vi "Create Gradient 32f.vi"(8 "Error In":errorcluster, 9 "Dimension":T1={"Depth"=1, "Height"=1, "Width"=1} {"Width" min=1; "Height" min=1; "Depth" min=1}, 11 "Device In":T4) -> (0 "Error Out":errorcluster, 1 "Dimension Out":T1={"Depth"=1, "Height"=1, "Width"=1} {"Width" min=1; "Height" min=1; "Depth" min=1}, 3 "Gradient Object":T2 {"Z"."Dimension"."Width" min=1; "Z"."Dimension"."Height" min=1; "Z"."Dimension"."Depth" min=1; "Y"."Dimension"."Width" min=1; "Y"."Dimension"."Height" min=1; "Y"."Dimension"."Depth" min=1; "X"."Dimension"."Width" min=1; "X"."Dimension"."Height" min=1; "X"."Dimension"."Depth" min=1})   [LabVIEW 2012, in "OpenCLV x64.lvlib"]
doc: "Creates a Gradient Object and allocates space for an X, Y, and Z destination memory objects."
uses:
  OpenCLV x64.lvlib
  Controls/Device ID.ctl
  User Controls/Array Dimensions.ctl
  Controls/Gradient Object.ctl
  Controls/Program Handle.ctl
  Controls/Memory Object.ctl
  Controls/Memory ID.ctl
  Controls/Memory Type.ctl
  Allocate Memory/AllocateMemory_32f.vi
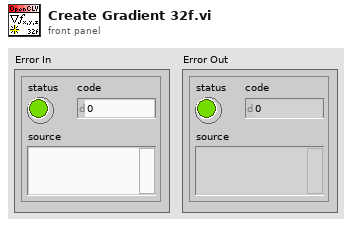
[diagram p1: front panel]
types:
  T1 = typedef "Array Dimensions.ctl" = cluster{"Depth":u64, "Height":u64, "Width":u64}
  T2 = typedef "OpenCLV x64.lvlib/Gradient Object.ctl" = cluster{"Program Handle":T3, "Device Out":T4, "X":T5, "Y":T5, "Z":T5}
  T3 = typedef "OpenCLV x64.lvlib/Program Handle.ctl" = u64
  T4 = typedef "OpenCLV x64.lvlib/Device ID.ctl" = u64
  T5 = typedef "OpenCLV x64.lvlib/Memory Object.ctl" = cluster{"Device ID":T4, "Memeroy ID":T6, "Dimension":T1, "Memory Type":T7}
  T6 = typedef "OpenCLV x64.lvlib/Memory ID.ctl" = u64
  T7 = typedef "OpenCLV x64.lvlib/Memory Type.ctl" = enum16{"32f", "u8", "i8", "u16", "i16", "u32", "i32", "64f"}
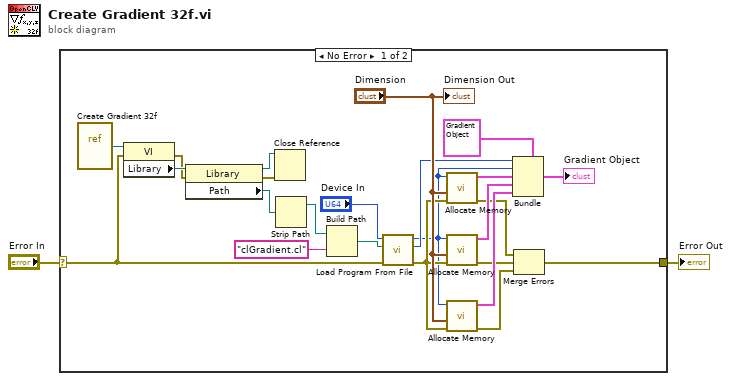
[diagram p0: block diagram]
diagram:
  n1 = case shown="No Error" "Error In" {
    selector: "Error In" -> [w3 w27]
    tunnel: [w16 w27] -> w1
    frame No Error {
      n2 = vi-ref "Create Gradient 32f.vi"() -> (w15:refnum<vi>)
      n3 = property class="VI"(reference=w15, error in=w3) -> (error out=w4:errorcluster, "Library"=w14:refnum<vi>)  [unwired: 1 out]
      n4 = property class="Library"(reference=w14, error in=w4) -> (reference out=w5:refnum<vi>, error out=w6:errorcluster, "Path"=w13:path)
      n5 = Close Reference(reference=w5, error in (no error)=w6) -> ()  [unwired: 1 out]
      n6 = Strip Path(path=w13) -> (stripped path=w26:path)  [unwired: 1 out]
      n7 = Build Path(base path=w26, name or relative path="clGradient.cl") -> (appended path=w24:path)
      n8 = call "Load Program From File.vi"("Error In"=w3, "Program Path"=w24, "Device In"="Device In") -> ("Error Out"=w21:errorcluster, "Program Handle"=w20:T3, "Device Out"=w19:T4)  [unwired: 6 in]
      n9 = call-poly "Allocate Memory.vi"("Error In"=w21, "Dimension"="Dimension", "Device In"=w19) -> ("Error Out"=w8:errorcluster, "Memory Object"=w7:T5)  [unwired: 6 in, 1 out]
      n10 = call-poly "Allocate Memory.vi"("Error In"=w21, "Dimension"="Dimension", "Device In"=w19) -> ("Error Out"=w10:errorcluster, "Memory Object"=w9:T5)  [unwired: 6 in, 1 out]
      n11 = call-poly "Allocate Memory.vi"("Error In"=w21, "Dimension"="Dimension", "Device In"=w19) -> ("Error Out"=w11:errorcluster, "Memory Object"=w12:T5)  [unwired: 6 in, 1 out]
      n12 = Bundle(cluster=T2 {"Program Handle"=0, "Device Out"=0, "X"={"Device ID"=0, "Memeroy ID"=0, "Dimension"={"Depth"=0, "Height"=0, "Width"=0}, "Memory Type"=enum."32f"}, "Y"={"Device ID"=0, "Memeroy ID"=0, "Dimension"={"Depth"=0, "Height"=0, "Width"=0}, "Memory Type"=enum."32f"}, "Z"={"Device ID"=0, "Memeroy ID"=0, "Dimension"={"Depth"=0, "Height"=0, "Width"=0}, "Memory Type"=enum."32f"}} ("output cluster"), "Program Handle"=w20, "Device Out"=w19, "X"=w7, "Y"=w9, "Z"=w12) -> (→"Gradient Object":T2)
      n13 = Merge Errors(w8, w10, w11) -> (w16:errorcluster)
      "Dimension Out" <- "Dimension"
    }
    frame Error {
    }
  }
  "Error Out" <- w1
